vi "PH_BeamlineController.Path set PA DP Target.vi"(0 "i ref in":refnum<vi>, 5 "error in (no error)":errorcluster) -> (14 "i ref out":refnum<vi>, 17 "Path changed?":bool, 19 "error out":errorcluster)   [LabVIEW 2014, in "PH_BeamlineController.lvlib"]
doc: "This VI writes incoming Information to own Attributes if the new value differs from the stored."
uses:
  PH_BeamlineController.lvlib
  PH_BeamlineController.PA DP Targets.ctl
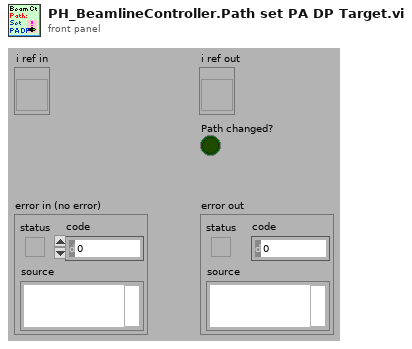
[diagram p1: front panel]
types:
  T1 = typedef "PH_BeamlineController.lvlib/PH_BeamlineController.PA DP Targets.ctl" = enum16{"None", "Dump PA Delayed Beam", "Dump PA Undelayed Beam", "Dumps PA Delayed and Undelayed Beam"}
  T2 = typedef "PH_BeamlineController.lvlib/PH_BeamlineController.PA DP Target Attributes.ctl" = cluster{"Name":T1, "GUI Ref":refnum<vi>, "Current State":bool, "Wanted State":bool, "Enabled":bool}
  T3 = typedef "PH_BeamlineController.lvlib/PH_BeamlineController.i attribute.ctl" = cluster{"Vacuum Exp LB":cluster{"Channel":string, "Limit [mbar]":dbl, "Pressure [mbar]":dbl, "GUI Ref":refnum<vi>}, "Sources":T4[], "PA DP Targets":T2[], "Path":cluster{"Source":T5, "PA DP Target":T1, "Target":T6}, "Targets":cluster{"Name":T6, "GUI Ref":refnum<vi>, "Current State":bool, "Wanted State":bool, "Enabled":bool}[], "Status Tags":cluster{"Name":string, "Status":T7}[], "special GUI Refs":T8}
  T4 = typedef "PH_BeamlineController.lvlib/PH_BeamlineController.Source Attributes.ctl" = cluster{"Name":T5, "GUI Ref":refnum<vi>, "Current State":bool, "Wanted State":bool}
  T5 = typedef "PH_BeamlineController.lvlib/PH_BeamlineController.Sources.ctl" = enum16{"None", "YLF", "fs-Frontend", "ns-Frontend", "YLF and ns-Frontend", "fs- and ns-Frontend"}
  T6 = typedef "PH_BeamlineController.lvlib/PH_BeamlineController.Targets.ctl" = enum16{"None", "PreAmp", "Dump Exp Laserlab", "Exp Laserlab", "Calorimeter", "Dump Exp Laserbay", "Exp Laserbay", "Dump Exp Z6", "Exp Z6"}
  T7 = typedef "PH_StatusHandler.lvlib/PH_StatusHandler.Status.ctl" = i16
  T8 = typedef "PH_BeamlineController.lvlib/PH_BeamlineController.special GUI Refs.ctl" = cluster{"PA-Backreflection-Meas":refnum<vi>, "fs_Synchrolock_Watch":refnum<vi>}
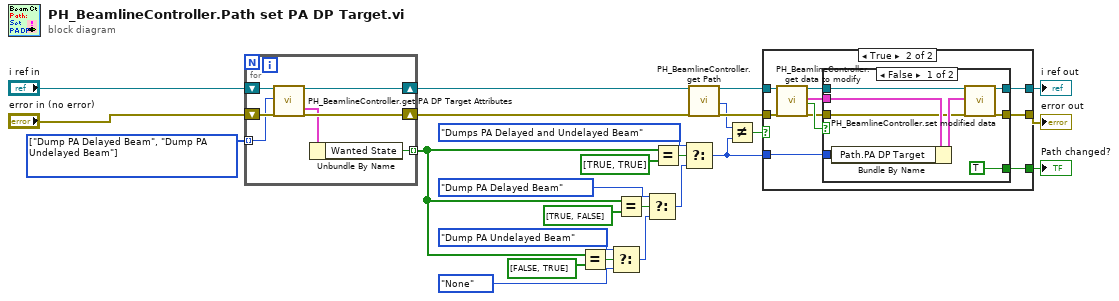
[diagram p0: block diagram]
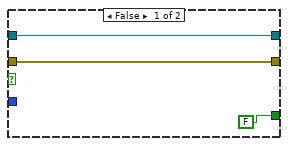
[diagram p2: hidden frame]
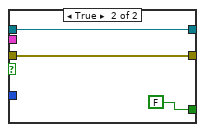
[diagram p3: hidden frame]
diagram:
  w15 = T1[] [enum."Dump PA Delayed Beam", enum."Dump PA Undelayed Beam"] items=["None", "Dump PA Delayed Beam", "Dump PA Undelayed Beam", "Dumps PA Delayed and Undelayed Beam"]
  n1 = for {
    shift-right: [w30] -> w17
    shift-left: "i ref in" -> [w32]
    shift-right: [w33] -> w20
    shift-left: "error in (no error)" -> [w31]
    tunnel: w15 -> [w29] mode=indexing
    tunnel: [w27] -> w1 mode=indexing
    n2 = call "PH_BeamlineController.get PA DP Target Attributes.vi"("VI in"=w32, "PA DP Target"=w29, "error in (no error)"=w31) -> ("VI out"=w30:refnum<vi>, "PA DP Target Attributes"=w28:T2, "error out"=w33:errorcluster)  [unwired: 13 in, 1 out]
    n3 = Unbundle By Name(w28) -> ("Wanted State"=w27:bool)
  }
  n4 = Equal?(x=w1, y=bool[] [FALSE, TRUE]) -> (x = y?=w6:bool)
  n5 = Select(t=PH_BeamlineController.PA_DP_Targets."Dump PA Undelayed Beam" ("SideTarget"), s=w6, f=PH_BeamlineController.PA_DP_Targets."None" ("SideTarget")) -> (s? t:f=w2:T1)
  n6 = Equal?(x=w1, y=bool[] [TRUE, FALSE]) -> (x = y?=w10:bool)
  n7 = Select(t=PH_BeamlineController.PA_DP_Targets."Dump PA Delayed Beam" ("SideTarget"), s=w10, f=w2) -> (s? t:f=w7:T1)
  n8 = Equal?(x=w1, y=bool[] [TRUE, TRUE]) -> (x = y?=w14:bool)
  n9 = Select(t=PH_BeamlineController.PA_DP_Targets."Dumps PA Delayed and Undelayed Beam" ("SideTarget"), s=w14, f=w7) -> (s? t:f=w11:T1)
  n10 = call "PH_BeamlineController.get Path.vi"("VI in"=w17, "error in (no error)"=w20) -> ("VI out"=w22:refnum<vi>, "Path:  PA DP Targets"=w16:T1, "error out"=w21:errorcluster)  [unwired: 12 in, 3 out]
  n11 = Not Equal?(x=w16, y=w11) -> (x != y?=w23:bool)
  n12 = case shown="True" w23 {
    tunnel: w11 -> [_ w46]
    tunnel: [w36 w41] -> w25
    tunnel: [w35 w40] -> w26
    tunnel: w21 -> [w35 w39]
    tunnel: w22 -> [w36 w38]
    tunnel: [FALSE w37] -> w24
    frame False {
    }
    frame True {
      n13 = call "PH_BeamlineController.get data to modify.vi"("i ref in"=w38, "error in (no error)"=w39) -> ("i ref out"=w42:refnum<vi>, "i attribute"=w44:T3, "timed out"=w45:bool, "error out"=w43:errorcluster)  [unwired: 14 in]
      n14 = case shown="False" w45 {
        tunnel: w42 -> [w50 w57]
        tunnel: [w54 w57] -> w41
        tunnel: w43 -> [w49 w56]
        tunnel: [w53 w56] -> w40
        tunnel: w44 -> [w52 _]
        tunnel: w46 -> [w47 _]
        tunnel: [TRUE FALSE] -> w37
        frame False {
          n15 = Bundle By Name(cluster=w52, "Path.PA DP Target"=w47) -> (w51:T3)
          n16 = call "PH_BeamlineController.set modified data.vi"("i ref in"=w50, "i attribute"=w51, "error in (no error)"=w49) -> ("i ref out"=w54:refnum<vi>, "error out"=w53:errorcluster)  [unwired: 15 in]
        }
        frame True {
        }
      }
    }
  }
  "error out" <- w26
  "i ref out" <- w25
  "Path changed?" <- w24
